vi "LineSettings(SubVI).vi"(6 "LVObjRef Refnum":refnum<vi>, 8 "Error In":errorcluster, 9 "element":T1 {"Color" format="%x"}, 10 "NumPlot":dbl, 11 "XYGraph in":refnum<vi>) -> (0 "Error Out":errorcluster)   [LabVIEW 2018]
uses:
  CTL/Line.ctl
  Windows/Settings/View.ctl
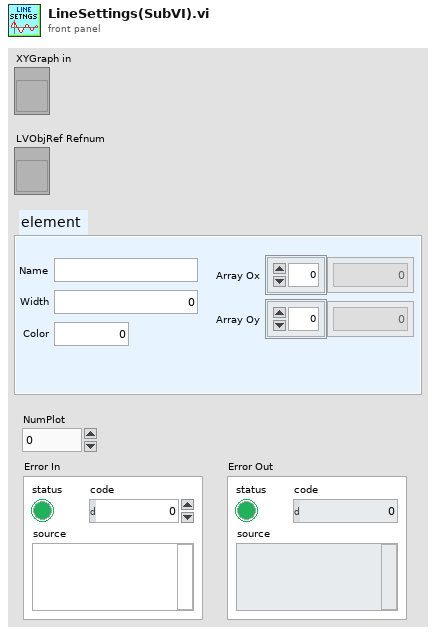
[diagram p1: front panel]
types:
  T1 = typedef "Line.ctl" = cluster{"Width":dbl, "Color":i64, "Array Oy":dbl[], "Array Ox":dbl[], "Name":string, "Plot Visible":T2}
  T2 = typedef "View.ctl" = bool
  T3 = typedef "LVComboBoxStrsAndValuesArrayTypeDef.ctl" = cluster{"String":string, "Value":string}[]
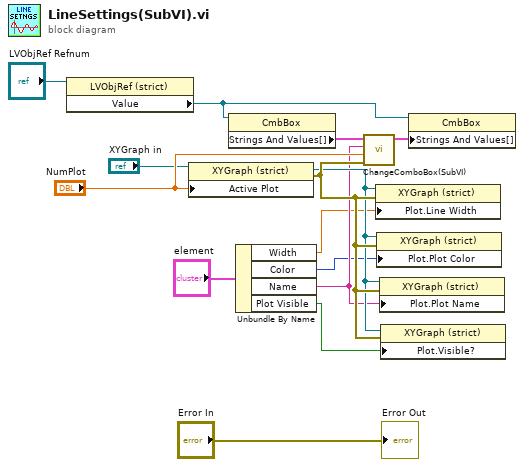
[diagram p0: block diagram]
diagram:
  n1 = property on="Property Node" class="LVObjRef (strict)"(reference="LVObjRef Refnum") -> ("Value"=w8:refnum<vi>)  [unwired: 1 in, 2 out]
  n2 = property on="Property Node" class="XYGraph (strict)"(reference="XYGraph in", "Active Plot"="NumPlot") -> (reference out=w11:refnum<vi>, error out=w13:errorcluster)  [unwired: 1 in]
  n3 = property on="Property Node" class="CmbBox"(reference=w8) -> ("Strings And Values[]"=w6:T3)  [unwired: 1 in, 2 out]
  n4 = Unbundle By Name("element") -> ("Width"=w3:dbl, "Color"=w5:i64, "Name"=w9:string, "Plot Visible"=w4:T2)
  n5 = call "ChangeComboBox(SubVI).vi"("Error In"=w13, "NumPlot"="NumPlot", "Name"=w9, "Strings and Values In[]"=w6) -> ("Strings and Values Out[]"=w7:cluster{"String":string, "Value":string}[])  [unwired: 6 in, 1 out]
  n6 = property on="Property Node" class="XYGraph (strict)"(reference=w11, error in=w13, "Plot.Line Width"=w3) -> ()  [unwired: 2 out]
  n7 = property on="Property Node" class="XYGraph (strict)"(reference=w11, error in=w13, "Plot.Plot Color"=w5) -> ()  [unwired: 2 out]
  n8 = property on="Property Node" class="XYGraph (strict)"(reference=w11, error in=w13, "Plot.Plot Name"=w9) -> ()  [unwired: 2 out]
  n9 = property on="Property Node" class="XYGraph (strict)"(reference=w11, error in=w13, "Plot.Visible?"=w4) -> ()  [unwired: 2 out]
  n10 = property on="Property Node" class="CmbBox"(reference=w8, "Strings And Values[]"=w7) -> ()  [unwired: 1 in, 2 out]
  "Error Out" <- "Error In"
